vi "RAMP_LAUDA.vi"(0 "pause":bool=TRUE, 1 "manual":i32, 2 "Array":dbl[](array[numeric]), 3 "T_man":dbl, 4 "Seq":dbl[](array[numeric])=[30.0, 50.0, 60.0, 30.0, 20.0], 5 "reset":bool, 6 "TimeParams":dbl[](array[numeric])=[1.0, 1.0, 1.0, 1.0, 1.0], 7 "shutdown":bool, 12 "treshold":dbl) -> (9 "T in":dbl, 10 "STEP":i32, 13 "T ext":dbl, 14 "params":i32[](array[numeric]), 15 "T control":dbl)   [LabVIEW 2015]
uses:
  x64/Debug/BERTTA.dll
panel:
  out "params2":i32
  out "params0":i32
  out "params1":i32
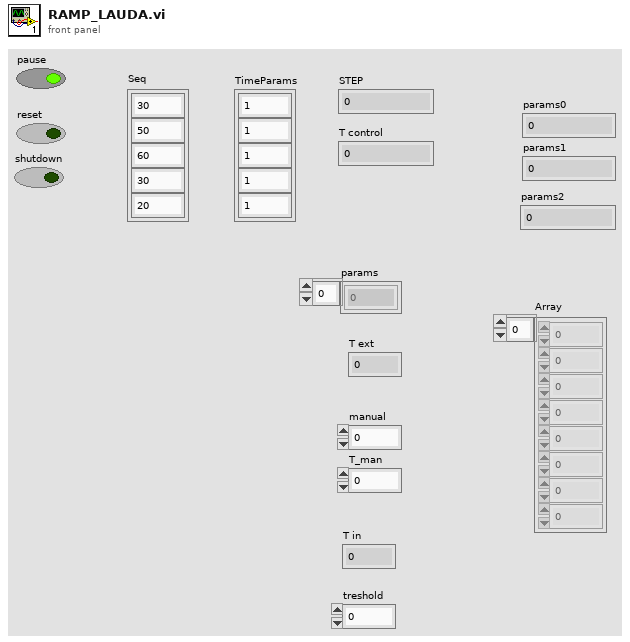
[diagram p1: front panel]
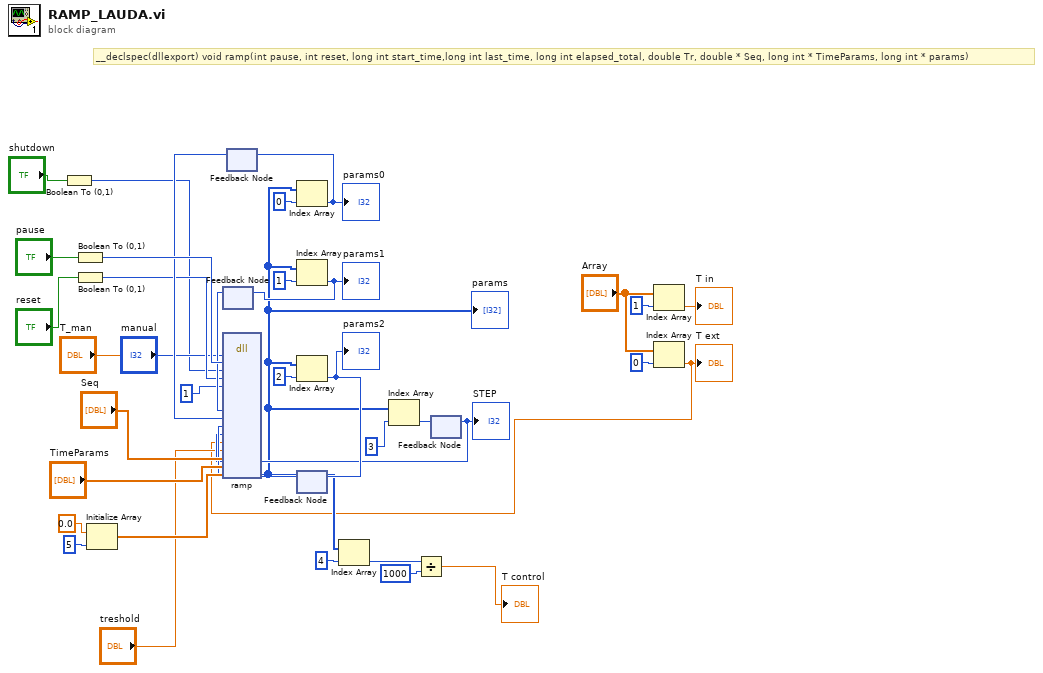
[diagram p0: block diagram]
diagram:
  # "__declspec(dllexport) void ramp(int pause, int reset, long int start_time,long int last_time, long int elapsed_total, double Tr, double * Seq, long int * TimeParams, long int * params)"
  n1 = Boolean To (0,1)(Boolean="shutdown") -> (0, 1=w6:i16)
  n2 = Boolean To (0,1)(Boolean="pause") -> (0, 1=w30:i16)
  n3 = Boolean To (0,1)(Boolean="reset") -> (0, 1=w24:i16)
  n4 = Initialize Array(0.0 ("element"), 5 ("dimension size")) -> (w37:dbl[])
  n5 = feedback #1() -> (w26:i32)  [unwired: 1 in]
  n6 = feedback #2() -> (w27:i32)  [unwired: 1 in]
  n7 = feedback #3() -> (w21:i32)  [unwired: 1 in]
  n8 = feedback #4() -> (w17:i32)  [unwired: 1 in]
  "STEP" <- w17
  n9 = Index Array(array="Array", index=1) -> (element=→"T in":dbl)
  n10 = Index Array(array="Array", index=0) -> (element=w1:dbl)
  "T ext" <- w1
  n11 = dll-call lib="C:/Users/shresplab/OneDrive - Kemira Oyj/Documents/Visual Studio 2017/Projects/Bertta/BERTTA/x64/Debug/BERTTA.dll" fn="ramp"("pause"=w30, "shutdown"=w6, "reset"=w24, "grad"=1, "manual"="manual", "T_man"="T_man", "start_time"=w26, "last_time"=w27, "elapsed_total"=w21, "step"=w17, "Tr"=w1, "treshold"="treshold", "Seq"="Seq", "TimeParams"="TimeParams", "params"=w37) -> ("params"=w15:i32[])  [unwired: 18 in, 2 out]
  "params" <- w15
  n12 = Index Array(array=w15, index=0) -> (element=w32:i32)
  "params0" <- w32
  n13 = feedback-in #2(w32) -> ()
  n14 = Index Array(array=w15, index=1) -> (element=w31:i32)
  "params1" <- w31
  n15 = feedback-in #1(w31) -> ()
  n16 = Index Array(array=w15, index=2) -> (element=w20:i32)
  "params2" <- w20
  n17 = feedback-in #3(w20) -> ()
  n18 = Index Array(array=w15, index=4) -> (element=w14:i32)
  n19 = Index Array(array=w15, index=3) -> (element=w18:i32)
  n20 = Divide(x=w14, y=1000) -> (x/y=→"T control":dbl)
  n21 = feedback-in #4(w18) -> ()
